vi "Actor Core.vi"(8 "error in (no error)":errorcluster, 11 "Mag Lab Measure Interface in":refnum<class "Mag Lab Measure UI.lvclass">) -> (0 "error out":errorcluster, 3 "Actor Framework.lvlib:Actor":refnum<class "Actor.lvclass">)   [LabVIEW 2015, in "Mag Lab Measure UI.lvclass"]
uses:
  Mag Lab Measure UI.lvclass
  <vilib>/ActorFramework/Actor/Actor.lvclass
  Mag Lab Measure UI.lvclass/Mag Lab Measure UI.ctl
  <vilib>/ActorFramework/Actor/Actor.lvclass/Actor.ctl
  <vilib>/ActorFramework/Message Enqueuer/Message Enqueuer.lvclass/Message Enqueuer.ctl
  Mag Lab Measure Interface Messages/Open menu object parameters Msg/Open menu object parameters Msg.lvclass/Open menu object parameters Msg.ctl
  <vilib>/ActorFramework/Message Enqueuer/Init from Existing Queue.vi
  <vilib>/ActorFramework/Message Enqueuer/Enqueue.vi
  <vilib>/ActorFramework/Message Priority Queue/Priority Enqueue.vi
  <vilib>/ActorFramework/Message Enqueuer/Message Enqueuer.lvclass
  <vilib>/ActorFramework/Stop Msg/Stop Msg.lvclass
  Mag Lab Measure Interface Messages/Open menu object parameters Msg/Open menu object parameters Msg.lvclass
  Mag Lab Root/Mag Lab Root.lvclass
  Mag Lab Error Handler/Mag Lab Error Handler.lvclass
panel:
  in  "No UI has been defined for this \nobject":bool
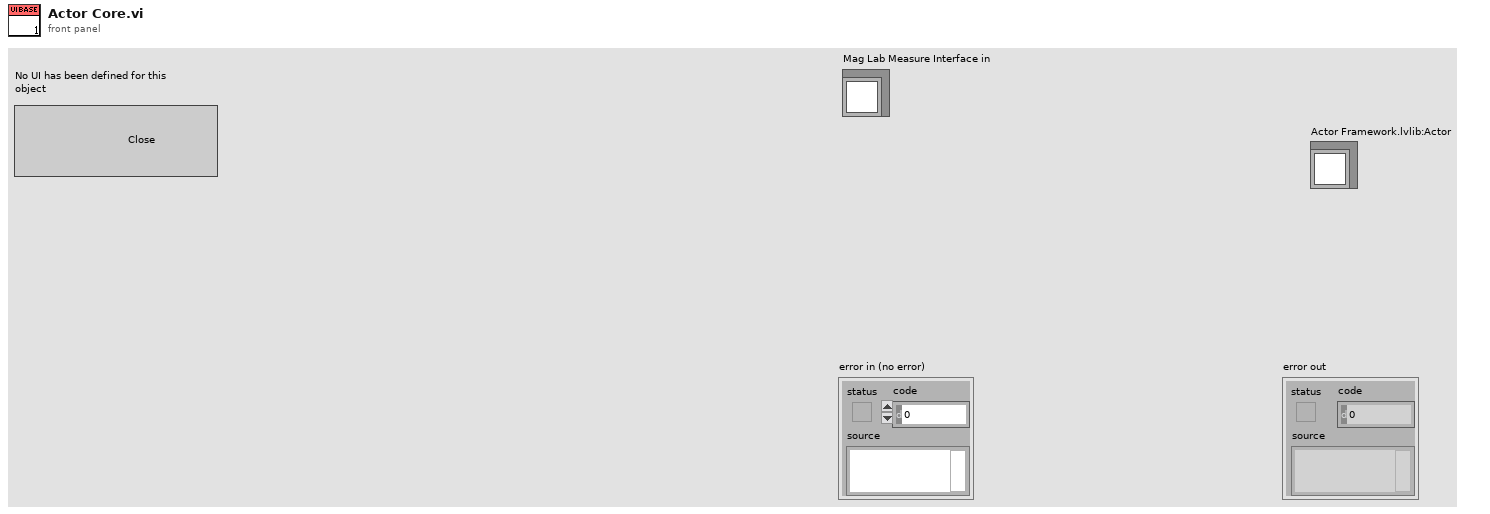
[diagram p1: front panel]
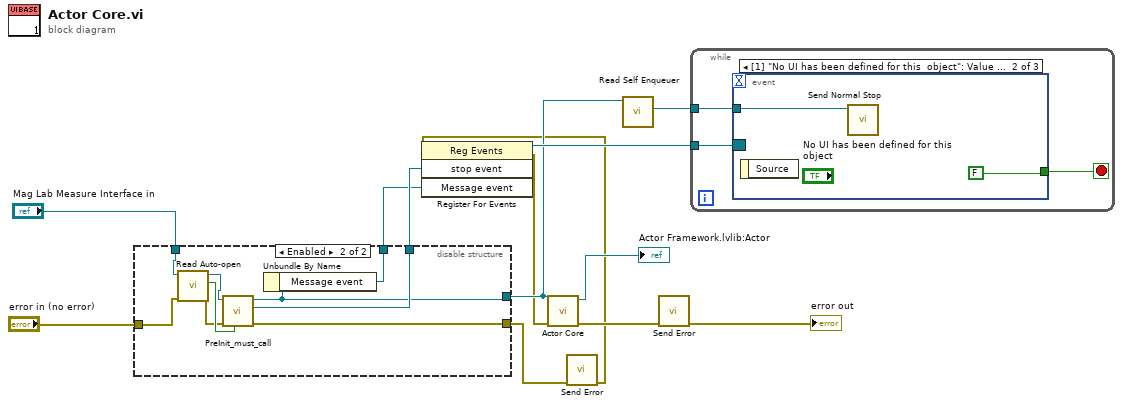
[diagram p0: block diagram]
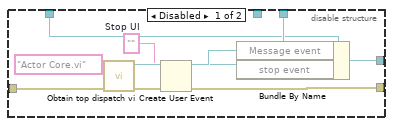
[diagram p2: hidden frame]
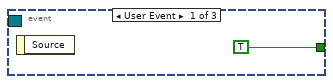
[diagram p3: hidden frame]
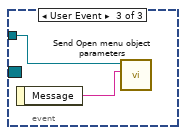
[diagram p4: hidden frame]
diagram:
  n1 = disable-structure shown="Enabled" {
    disable-tunnel: "error in (no error)" -> [w21 w23]
    disable-tunnel: [w18 w28] -> w2
    disable-tunnel: [w16 w31] -> w10
    disable-tunnel: "Mag Lab Measure Interface in" -> [w15 w27]
    disable-tunnel: [w14 w30] -> w7
    disable-tunnel: [_ w29] -> w6
    frame Disabled {
      w17 = ""  # Stop UI
      n2 = call "Obtain top dispatch vi.vi"("Error In"=w21, "VI name"="Actor Core.vi") -> ("Error Out"=w19:errorcluster, "vi reference"=w20:refnum<vi>)  [unwired: 7 in, 1 out]
      n3 = Create User Event(user event datatype=w17, error in=w19) -> (user event=w16:refnum<user-event>, error out=w18:errorcluster)
      n4 = Bundle By Name(cluster=w15, "Message event"=w20, "stop event"=w16) -> (w14:refnum<class "Mag Lab Measure UI.lvclass">)
    }
    frame Enabled {
      n5 = call "Read Auto-open.vi"("error in (no error)"=w23, "Mag Lab Measure UI in"=w27) -> ("error out"=w24:errorcluster, "Auto-open"=w26:bool, "Mag Lab Measure UI out"=w25:refnum<class "Mag Lab Measure UI.lvclass">)  [unwired: 7 in]
      n6 = call-dynamic "PreInit_must_call.vi"("Open Actor Core front panel? (T)"=w26, "error in (no error)"=w24, "Mag Lab Measure Interface in"=w25) -> ("error out"=w28:errorcluster, "stop event"=w31:refnum<user-event>, "Mag Lab Measure Interface out"=w30:refnum<class "Mag Lab Measure UI.lvclass">)  [unwired: 6 in]
      n7 = Unbundle By Name(w30) -> ("Message event"=w29:refnum<user-event>)
    }
  }
  n8 = call "Send Error.vi"("error in (no error)"=w2) -> ("error out"=w1:errorcluster)  [unwired: 9 in, 1 out]
  n9 = register-events(error in=w1, w10, w6) -> (reference out=w11:refnum<event-registration>, error out=w5:errorcluster)  [unwired: 1 in]
  n10 = call-parent "Actor Core.vi"("error in"=w5, "Actor in"=w7) -> ("error out"=w4:errorcluster, "Actor out"=→"Actor Framework.lvlib:Actor":refnum<class "Actor.lvclass">)  [unwired: 8 in]
  n11 = call <vilib>:"Read Self Enqueuer.vi"("Actor"=w7) -> ("Self Enqueuer"=w8:refnum<class "Message Enqueuer.lvclass">)  [unwired: 10 in]
  n12 = call "Send Error.vi"("error in (no error)"=w4) -> ("error out"=→"error out":errorcluster)  [unwired: 9 in, 1 out]
  n13 = while {
    tunnel: w11 -> [w33]
    tunnel: w8 -> [w32]
    stop <- w34 stop-if-true
    n14 = event shown="[1] \"No UI has been defined for this  object\": Value Change" {
      selector: w33 -> [_ _ _]
      dyn-events: _ -> [_ _ _]
      timeout: _ -> [_ _ _]
      tunnel: [TRUE FALSE _] -> w34
      tunnel: w32 -> [_ w37 w39]
      event User Event {
        n15 = event-data() -> ()  [unwired: 1 in, 1 out]
      }
      event "No UI has been defined for this \nobject": Value Change {
        n16 = event-data() -> ()  [unwired: 1 in, 1 out]
        n17 = call <vilib>:"Send Normal Stop.vi"("Message Enqueuer"=w37) -> ()  [unwired: 10 in, 1 out]
      }
      event User Event {
        n18 = event-data() -> ("Message"=w38:string)  [unwired: 1 in]
        n19 = call "Send Open menu object parameters.vi"("Object name"=w38, "Message Enqueuer"=w39) -> ()  [unwired: 8 in, 2 out]
      }
    }
  }
